vi "send request, get response.vi"(8 "error in (no error)":errorcluster, 10 "request":string, 11 "zmq_socket in":refnum<class "zmq_socket.lvclass">) -> (0 "error out":errorcluster, 1 "response":string, 2 "timeout?":bool, 3 "zmq_socket out":refnum<class "zmq_socket.lvclass">, 5 "more?":bool)   [LabVIEW 2018, in "LV2Julia_core.lvlib"]
uses:
  <vilib>/addons/zeromq/zmq_socket.lvclass
  LV2Julia_core.lvlib
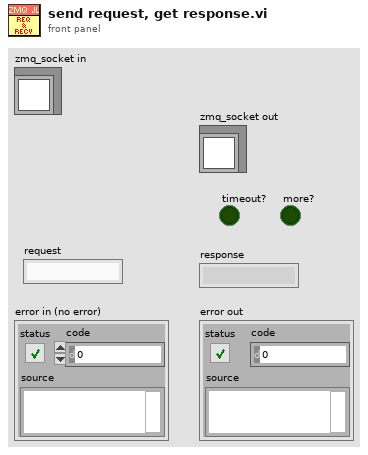
[diagram p1: front panel]
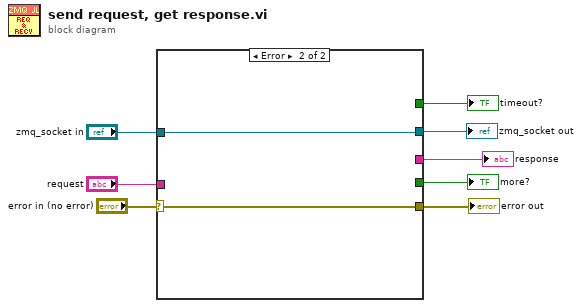
[diagram p0: block diagram]
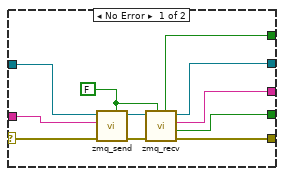
[diagram p2: hidden frame]
diagram:
  n1 = case shown="Error" "error in (no error)" {
    selector: "error in (no error)" -> [w9 w21]
    tunnel: [w19 _] -> w8
    tunnel: [w18 _] -> w7
    tunnel: [w16 _] -> w6
    tunnel: "request" -> [w15 _]
    tunnel: [w13 w20] -> w4
    tunnel: [w12 w21] -> w3
    tunnel: "zmq_socket in" -> [w10 w20]
    frame No Error {
      w17 = FALSE ("more? (F)")
      n2 = call <vilib>:"zmq_send.vi"("error in"=w9, "data"=w15, "socket in"=w10, "more? (F)"=w17) -> ("error out"=w14:errorcluster, "socket out"=w11:refnum<class "zmq_socket.lvclass">)  [unwired: 3 in]
      n3 = call <vilib>:"zmq_recv.vi"("no block? (F)"=w17, "error in"=w14, "socket in"=w11) -> ("error out"=w12:errorcluster, "more?"=w19:bool, "data"=w16:string, "socket out"=w13:refnum<class "zmq_socket.lvclass">, "timeout?"=w18:bool)  [unwired: 2 in]
    }
    frame Error {
    }
  }
  "more?" <- w8
  "timeout?" <- w7
  "response" <- w6
  "zmq_socket out" <- w4
  "error out" <- w3
